vi "Read and Write Controls to File.vi"(7 "Action":T1, 8 "error in":errorcluster, 9 "Control References":refnum<vi>[](array[refnum]), 11 "configuration file path":path) -> (0 "error out":errorcluster)   [LabVIEW 2015]
uses:
  Load and Save Controls_LV2009.llb/RWC_Actions.ctl
  <vilib>/Utility/config.llb/NI_LVConfig.lvlib
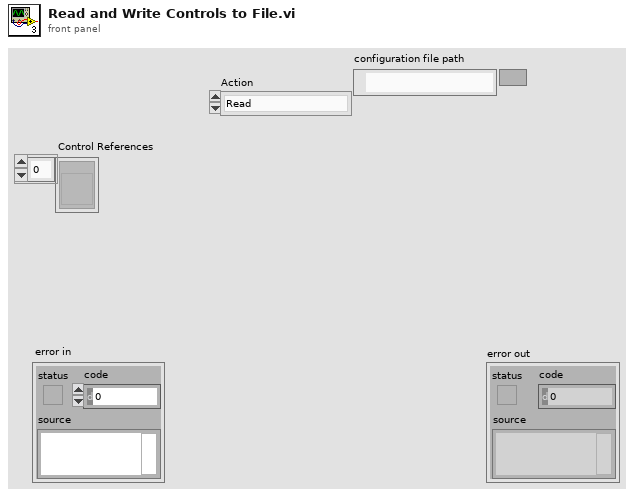
[diagram p1: front panel]
types:
  T1 = typedef "RWC_Actions.ctl" = enum16{"Read", "Write", "Read and Create"}
  T2 = typedef "NI_LVConfig.lvlib/Config Data RefNum.ctl" = refnum<k1>
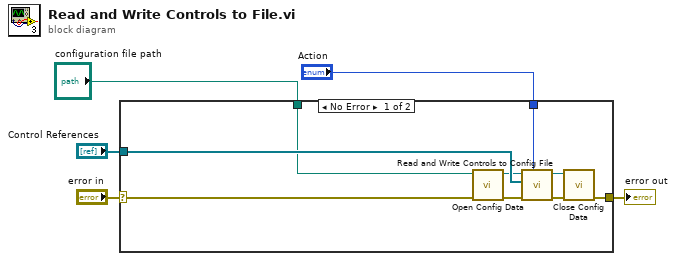
[diagram p0: block diagram]
diagram:
  n1 = case shown="No Error" "error in" {
    selector: "error in" -> [w7 w15]
    tunnel: "Action" -> [w14 _]
    tunnel: "Control References" -> [w13 _]
    tunnel: [w8 w15] -> w2
    tunnel: "configuration file path" -> [w6 _]
    frame No Error {
      n2 = call <vilib>:"Open Config Data.vi"("error in (no error)"=w7, "configuration file path"=w6) -> ("error out"=w12:errorcluster, "refnum"=w10:T2)  [unwired: 7 in, 1 out]
      n3 = call "Read and Write Controls to Config File.vi"("Action"=w14, "error in"=w12, "Control References"=w13, "Configuration File Reference In"=w10) -> ("error out"=w9:errorcluster, "Configuration File Reference Out"=w11:T2)  [unwired: 6 in]
      n4 = call <vilib>:"Close Config Data.vi"("error in (no error)"=w9, "refnum"=w11) -> ("error out"=w8:errorcluster)  [unwired: 8 in, 1 out]
    }
    frame Error {
    }
  }
  "error out" <- w2
